vi "Osciloscopio.vi"() -> ()   [LabVIEW 2016]
uses:
  <instrlib>/Tektronix TDS 200 1000 2000 Series/Public/Data/Read (Multiple Waveforms).vi
  <instrlib>/Tektronix TDS 200 1000 2000 Series/Tektronix TDS 200 1000 2000 Series.lvlib
panel:
  out "Waveform Data":waveform(dbl)[](graph)
  in  "VISA resource name":refnum<visa-resource-name>
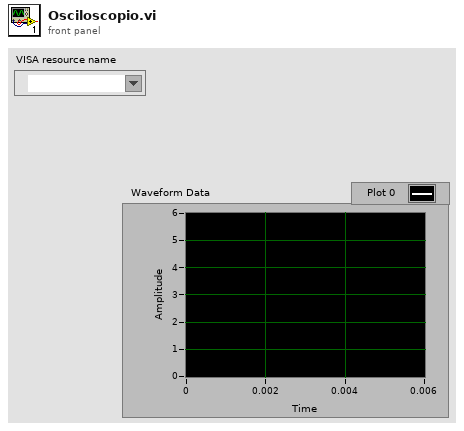
[diagram p1: front panel]
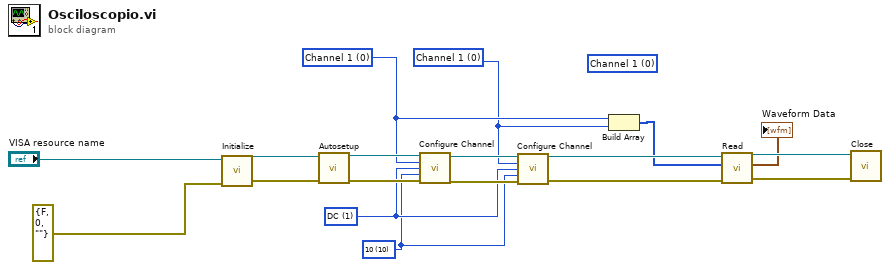
[diagram p0: block diagram]
diagram:
  w6 = 10 items=["1"=1, "10"=10, "20"=20, "50"=50, "100"=100, "500"=500, "1000"=1000] ("Probe Attenuation (10: 10X)")
  w7 = 1 items=["AC", "DC", "Ground"] ("Vertical Coupling (1: DC)")
  w4 = 0 items=["Channel 1", "Channel 2", "Channel 3", "Channel 4", "Math", "Reference A", "Reference B", "Reference C", "Reference D"] ("Channel (0: Channel 1)")
  w5 = 0 items=["Channel 1", "Channel 2", "Channel 3", "Channel 4", "Math", "Reference A", "Reference B", "Reference C", "Reference D"] ("Channel (0: Channel 1)")
  (unwired) u16 0 items=["Channel 1", "Channel 2", "Channel 3", "Channel 4", "Math", "Reference A", "Reference B", "Reference C", "Reference D", "FFT"] ("Source (0: Channel 1)")
  n1 = call <instrlib>:"Initialize.vi"("error in (no error)"=errorcluster {"status"=FALSE, "code"=0, "source"=""}, "VISA resource name"="VISA resource name") -> ("error out"=w15:errorcluster, "VISA resource name out"=w16:refnum<visa-resource-name>)  [unwired: 8 in]
  n2 = call <instrlib>:"Autosetup.vi"("error in (no error)"=w15, "VISA resource name"=w16) -> ("error out"=w10:errorcluster, "VISA resource name out"=w11:refnum<visa-resource-name>)  [unwired: 8 in]
  n3 = call <instrlib>:"Configure Channel.vi"("VISA resource name"=w11, "Channel (0: Channel 1)"=w5, "Vertical Coupling (1: DC)"=w7, "Probe Attenuation (10: 10X)"=w6, "error in (no error)"=w10) -> ("VISA resource name out"=w9:refnum<visa-resource-name>, "error out"=w8:errorcluster)  [unwired: 9 in]
  n4 = call <instrlib>:"Configure Channel.vi"("VISA resource name"=w9, "Channel (0: Channel 1)"=w4, "Vertical Coupling (1: DC)"=w7, "Probe Attenuation (10: 10X)"=w6, "error in (no error)"=w8) -> ("VISA resource name out"=w3:refnum<visa-resource-name>, "error out"=w2:errorcluster)  [unwired: 9 in]
  n5 = Build Array(w5, w4) -> (w1:i32[])
  n6 = call-poly <instrlib>:"Read.vi"("error in (no error)"=w2, "Channels"=w1, "VISA resource name"=w3) -> ("error out"=w13:errorcluster, "Waveform Data"=→"Waveform Data":waveform(dbl)[], "VISA resource name out"=w14:refnum<visa-resource-name>)  [unwired: 6 in]
  n7 = call <instrlib>:"Close.vi"("error in (no error)"=w13, "VISA resource name"=w14) -> ()  [unwired: 9 in, 1 out]
